vi "Function for Xbox Deadzone.vi"(11 "input variable":dbl) -> (3 "output variable":dbl)   [LabVIEW 2014]
uses:
  <vilib>/gmath/NI_Gmath.lvlib
panel:
  in  "b":dbl
  in  "m":dbl
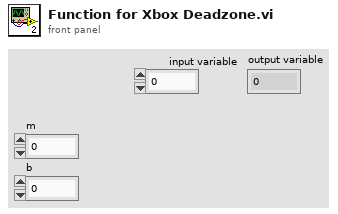
[diagram p1: front panel]
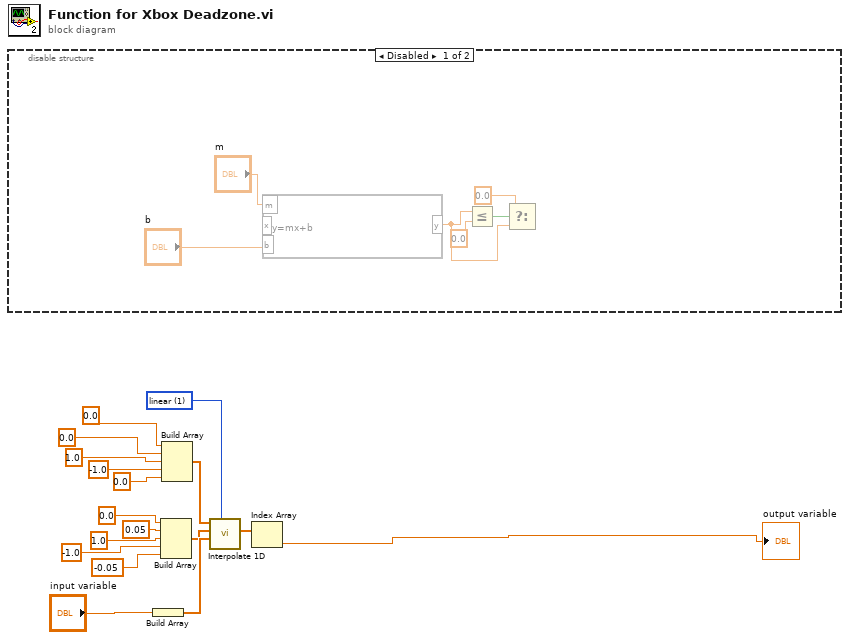
[diagram p0: block diagram]
diagram:
  w10 = 1 items=["nearest", "linear", "spline", "cubic Hermite", "Lagrange"] ("method")
  n1 = disable-structure shown="Disabled" {
    frame Disabled {
      n2 = formula code="y=mx+b"("m"="m", "b"="b") -> ("x"=w18:dbl, "y"=w20:dbl)
      n3 = Less Or Equal?(x=w20, y=0.0) -> (x <= y?=w22:bool)
      n4 = Select(t=0.0, s=w22, f=w20) -> (s? t:f=w19:dbl)
    }
    frame Enabled {
    }
  }
  n5 = Build Array("input variable") -> (w17:dbl[])
  n6 = Build Array(0.0 ("element"), 0.05 ("element"), 1.0 ("element"), -1.0 ("element"), -0.05 ("element")) -> (w12:dbl[])
  n7 = Build Array(0.0 ("element"), 0.0 ("element"), 1.0 ("element"), -1.0 ("element"), 0.0 ("element")) -> (w11:dbl[])
  n8 = call <vilib>:"Interpolate 1D.vi"("method"=w10, "xi"=w17, "X"=w12, "Y"=w11) -> ("xi used"=w9:dbl[])  [unwired: 5 in, 2 out]
  n9 = Index Array(array=w9) -> (element=→"output variable":dbl)  [unwired: 1 in]
